vi "FormatData.vi"(11 "Raw data":u64[](array[numeric])) -> (3 "Scaled":dbl[][](array[numeric]))   [LabVIEW 2018, in "FpgaRef5761.lvclass"]
uses:
  FpgaRef5761.lvclass
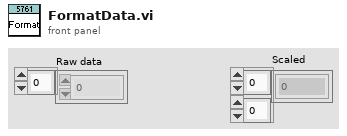
[diagram p1: front panel]
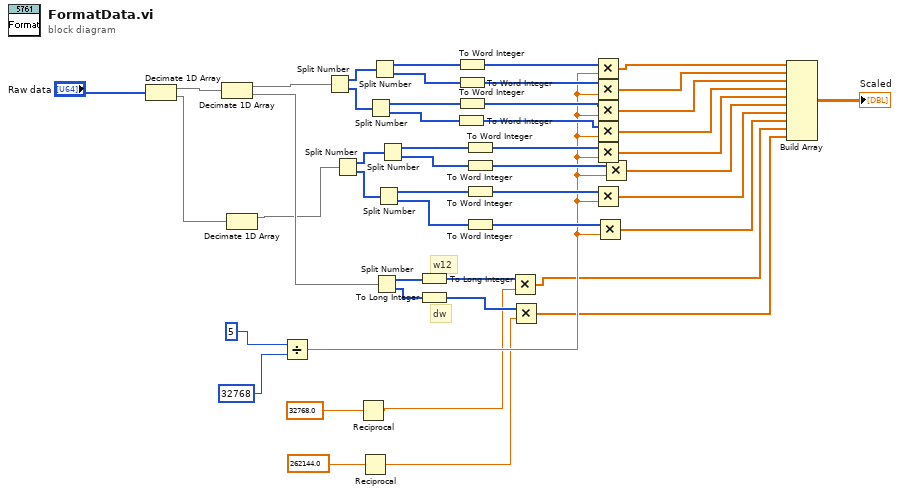
[diagram p0: block diagram]
diagram:
  # "dw"
  # "w12"
  n1 = Decimate 1D Array("Raw data") -> (w16:u64[], w15:u64[])
  n2 = Decimate 1D Array(w16) -> (w44:u64[], w8:u64[])
  n3 = Decimate 1D Array(w15) -> (w7:u64[])  [unwired: 1 out]
  n4 = Divide(x=5, y=32768) -> (x/y=w21:dbl)
  n5 = Split Number(x=w44) -> (hi(x)=w19:u32[], lo(x)=w20:u32[])
  n6 = Split Number(x=w7) -> (hi(x)=w18:u32[], lo(x)=w17:u32[])
  n7 = Reciprocal(x=32768.0) -> (1/x=w4:dbl)
  n8 = Reciprocal(x=262144.0) -> (1/x=w3:dbl)
  n9 = Split Number(x=w20) -> (hi(x)=w47:u16[], lo(x)=w46:u16[])
  n10 = Split Number(x=w19) -> (hi(x)=w45:u16[], lo(x)=w48:u16[])
  n11 = Split Number(x=w8) -> (hi(x)=w14:u32[], lo(x)=w13:u32[])
  n12 = Split Number(x=w17) -> (hi(x)=w41:u16[], lo(x)=w42:u16[])
  n13 = Split Number(x=w18) -> (hi(x)=w43:u16[], lo(x)=w40:u16[])
  n14 = To Long Integer(number=w14) -> (32bit integer=w12:i32[])
  n15 = To Long Integer(number=w13) -> (32bit integer=w11:i32[])
  n16 = To Word Integer(number=w46) -> (16bit integer=w35:i16[])
  n17 = To Word Integer(number=w45) -> (16bit integer=w38:i16[])
  n18 = To Word Integer(number=w48) -> (16bit integer=w37:i16[])
  n19 = To Word Integer(number=w47) -> (16bit integer=w36:i16[])
  n20 = To Word Integer(number=w43) -> (16bit integer=w34:i16[])
  n21 = To Word Integer(number=w40) -> (16bit integer=w33:i16[])
  n22 = To Word Integer(number=w41) -> (16bit integer=w32:i16[])
  n23 = To Word Integer(number=w42) -> (16bit integer=w31:i16[])
  n24 = Multiply(x=w12, y=w4) -> (x*y=w10:dbl[])
  n25 = Multiply(x=w11, y=w3) -> (x*y=w9:dbl[])
  n26 = Multiply(x=w38, y=w21) -> (x*y=w30:dbl[])
  n27 = Multiply(x=w37, y=w21) -> (x*y=w29:dbl[])
  n28 = Multiply(x=w36, y=w21) -> (x*y=w28:dbl[])
  n29 = Multiply(x=w35, y=w21) -> (x*y=w27:dbl[])
  n30 = Multiply(x=w34, y=w21) -> (x*y=w26:dbl[])
  n31 = Multiply(x=w32, y=w21) -> (x*y=w24:dbl[])
  n32 = Multiply(x=w31, y=w21) -> (x*y=w23:dbl[])
  n33 = Multiply(x=w33, y=w21) -> (x*y=w25:dbl[])
  n34 = Build Array(w30, w29, w28, w27, w26, w25, w24, w23, w10, w9) -> (→"Scaled":dbl[][])
